vi "Datasheet Yield.vi"(6 "Connection Refnum":T3, 8 "error in (no error)":errorcluster, 9 "Grouped Results":cluster{"Result Group":T1[]}[](array[cluster]), 10 "sxTemplateId":string, 11 "Parameters":T2) -> (0 "error out":errorcluster, 3 "report":path)   [LabVIEW 2011]
uses:
  SI.LIB/ODBC/SQL Controls/Connection Refnum.ctl
  Addons/internet/utils/keyedarr.llb/Keyed Array.ctl
  www/cgi-bin/_cgi-lib/TDM_INDEX Record.ctl
  Addons/internet/utils/strutil.llb/Case Matching.ctl
  Datasheet Analysis Parameters.ctl
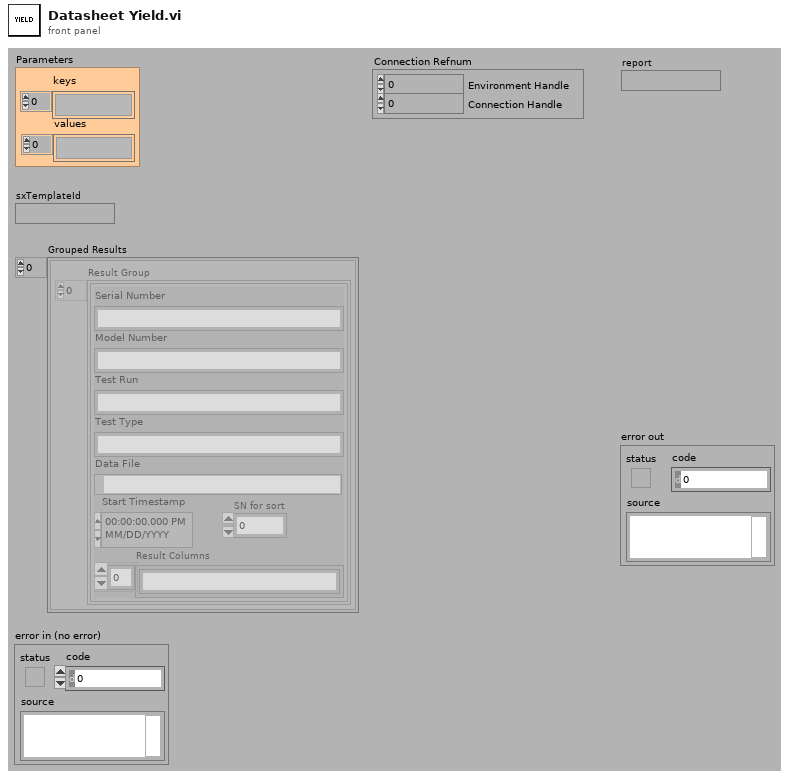
[diagram p1: front panel]
types:
  T1 = typedef "TDM_INDEX Record.ctl" = cluster{"Model Number":string, "SN for sort":i32, "Test Type":string, "Test Run":string, "Serial Number":string, "Start Timestamp":timestamp, "Data File":path, "Result Columns":string[]}
  T2 = typedef "Keyed Array.ctl" = cluster{"keys":string[], "values":string[]}
  T3 = typedef "Connection Refnum.ctl" = cluster{"Environment Handle":i32, "Connection Handle":i32}
  T4 = typedef "Datasheet Analysis Parameters.ctl" = cluster{"Test Type":string, "Parameter":string, "Sxx Format":string, "PIM Unit":string, "Start Frequency":dbl, "Stop Frequency":dbl, "Sort Property":string, "Show Raw?":bool, "Bin format":string, "Bin Type":string, "Bin_var":string}
  T5 = typedef "Case Matching.ctl" = enum16{"a != A", "a == A", "system"}
  T6 = typedef "CGI Yield Results.ctl" = cluster{"Model Number":string, "Serial Number for Sort":i32, "Serial Number":string, "Test Status":string, "Time Stamp":timestamp, "OperatorID":string, "Retry":i32, "First Pass?":bool}
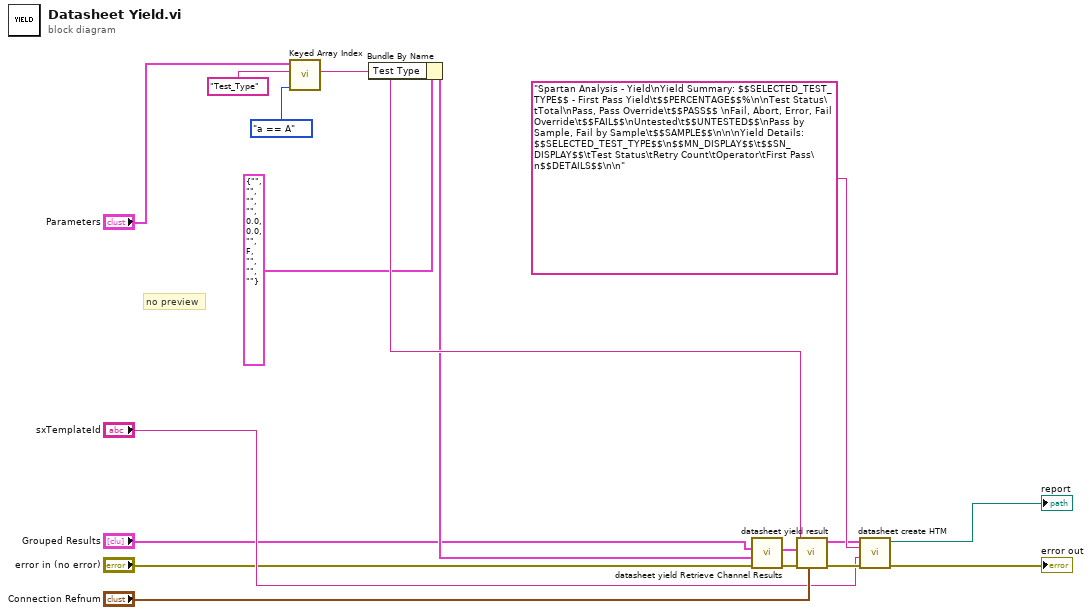
[diagram p0: block diagram]
diagram:
  # "no preview"
  n1 = call "Keyed Array Index.vi"("case matching (sensitive)"=Case_Matching."a == A", "key"="Test_Type" ("format string"), "array in"="Parameters") -> ("value"=w16:string)  [unwired: 1 in, 3 out]
  n2 = Bundle By Name(cluster=T4 {"Test Type"="", "Parameter"="", "Sxx Format"="", "PIM Unit"="", "Start Frequency"=0.0, "Stop Frequency"=0.0, "Sort Property"="", "Show Raw?"=FALSE, "Bin format"="", "Bin Type"="", "Bin_var"=""} ("Test Parameters"), "Test Type"=w16) -> (w9:T4)
  n3 = call "datasheet yield Retrieve Channel Results.vi"("error in (no error)"="error in (no error)", "Test Parameters"=w9, "Grouped Results"="Grouped Results") -> ("error out"=w13:errorcluster, "Array"=w11:T6[])  [unwired: 7 out]
  n4 = call "datasheet yield result.vi"("Connection Refnum"="Connection Refnum", "error in (no error)"=w13, "Yield Results"=w11, "Selected Test Type"=w16) -> ("error out"=w14:errorcluster, "Key Array Out"=w15:T2)  [unwired: 6 out]
  n5 = call "datasheet create HTM.vi"("error in (no error)"=w14, "sxTemplateId"="sxTemplateId", "template"="Spartan Analysis - Yield\nYield Summary: $$SELECTED_TEST_TYPE$$ - First Pass Yield\t$$PERCENTAGE$$%\n\nTest Status\tTotal\nPass, Pass Override\t$$PASS$$ \nFail, Abort, Error, Fail Override\t$$FAIL$$\nUntested\t$$UNTESTED$$\nPass by Sample, Fail by Sample\t$$SAMPLE$$\n\n\nYield Details: $$SELECTED_TEST_TYPE$$\n$$MN_DISPLAY$$\t$$SN_DISPLAY$$\tTest Status\tRetry Count\tOperator\tFirst Pass\n$$DETAILS$$\n\n", "array out"=w15) -> ("error out"=→"error out":errorcluster, "report"=→"report":path)  [unwired: 6 out]
